vi "Exemple_Preprocessing_QuantileTransformer.vi"() -> ()   [LabVIEW 2020]
uses:
  Objet/6 - Datasets Transformation/6.3 - Processing Data/QuantileTransformer/QuantileTransformer.lvclass
panel:
  in  "y":string[][](array[string])
  in  "X":string[][](array[string])=[["1", "2"], ["3", "4"], ["5", "6"], ["7", "8"], ["9", "10"]]
  out "Data":T1
  out "error out":errorcluster
  in  "error in":errorcluster caption="entrée d'erreur"
  in  "QuantileTransformer":T2={"n_quantiles"=10, "output_distribution"="uniform", "ignore_implicit_zeros"=FALSE, "subsample"=100000.0, "random_state"=0, "copy"=TRUE} {"random_state" min=-1}
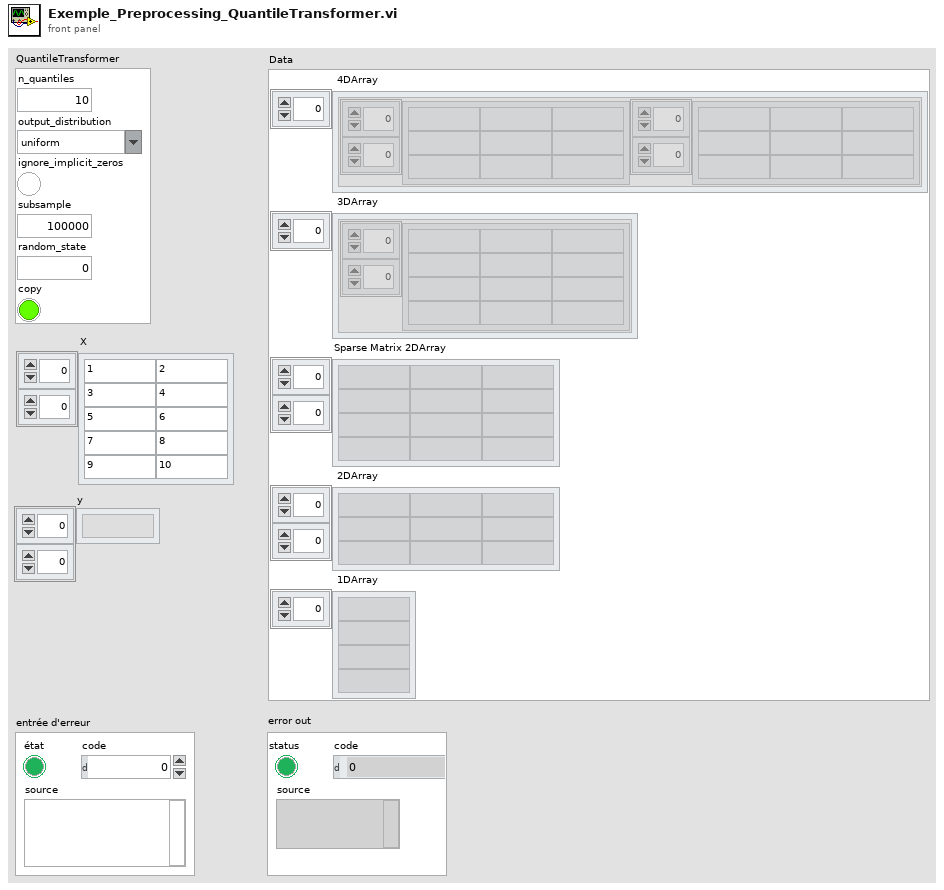
[diagram p1: front panel]
types:
  T1 = cluster{" 4DArray":cluster{"1":string[][], "2":string[][]}[], " 3DArray":cluster{"Tableau":string[][]}[], "Sparse Matrix 2DArray":string[][], " 2DArray":string[][], " 1DArray":string[]}
  T2 = cluster{"n_quantiles":i32, "output_distribution":string, "ignore_implicit_zeros":bool, "subsample":dbl, "random_state":i32, "copy":bool}
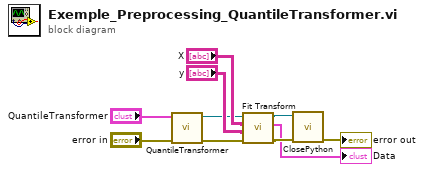
[diagram p0: block diagram]
diagram:
  n1 = call "QuantileTransformer.vi"("error in (no error)"="error in", "QuantileTransformer"="QuantileTransformer") -> ("error out"=w3:errorcluster, "QuantileTransformer.lvclass"=w4:refnum<class "QuantileTransformer.lvclass">)  [unwired: 8 in]
  n2 = call-dynamic "Fit Transform.vi"("error in (no error)"=w3, "y"="y", "X"="X", "QuantileTransformer.lvclass"=w4) -> ("error out"=w6:errorcluster, "Data"=→"Data":T1, "QuantileTransformer.lvclass"=w7:refnum<class "QuantileTransformer.lvclass">)  [unwired: 5 in]
  n3 = call-dynamic "ClosePython.vi"("error in (no error)"=w6, "Scikit-learn en entrée"=w7) -> ("error out"=→"error out":errorcluster)  [unwired: 8 in, 1 out]
